vi "Main.vi"() -> ()   [LabVIEW 2018]
uses:
  <vilib>/addons/zeromq/zmq_context.lvclass
  Channel Rep/Channel Rep.lvclass
  C:/Users/orlando/Documents/Orlando/communication-manager/communication-manager/Communication Channel/Communication Channel.lvclass
  Channel Req/Channel Req.lvclass
  Channel Sub/Channel Sub.lvclass
  Channel Pub/Channel Pub.lvclass
  Communication Channel/Communication Channel.lvclass
panel:
  in  "Channel Pub.lvclass":refnum<class "Channel Pub.lvclass">
  in  "Channel Sub.lvclass":refnum<class "Channel Sub.lvclass">
  in  "Channel Req.lvclass":refnum<class "Channel Req.lvclass">
  in  "Channel Rep.lvclass":refnum<class "Channel Rep.lvclass">
  out "context":refnum<class "zmq_context.lvclass">
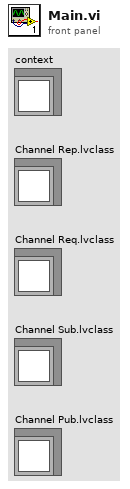
[diagram p1: front panel]
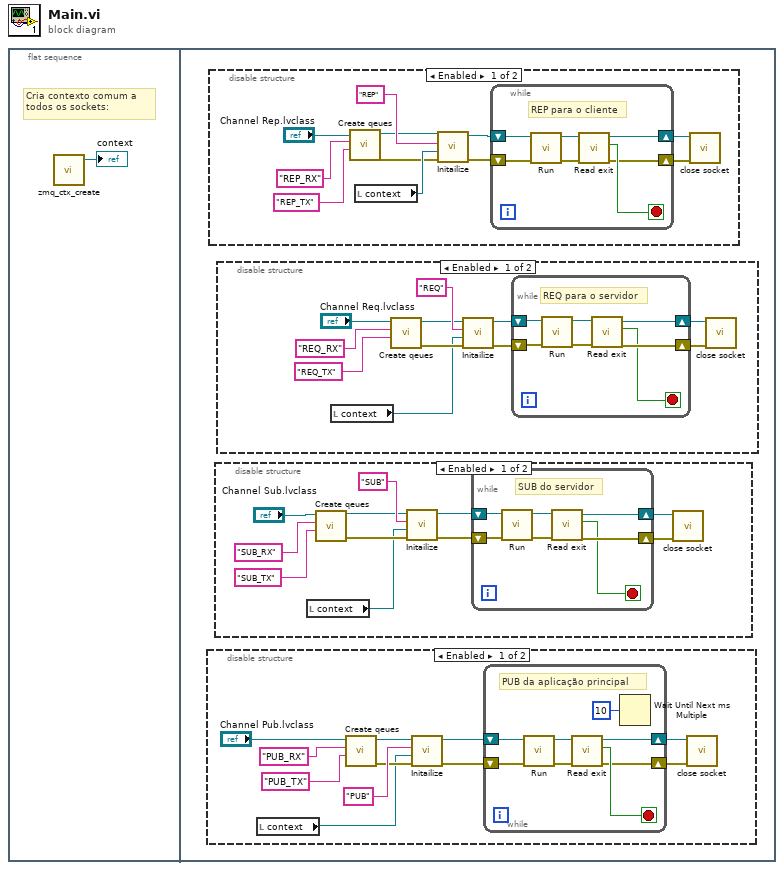
[diagram p0: block diagram]
diagram:
  n1 = flat-sequence {
    frame #0 {
      # "Cria contexto comum a \ntodos os sockets:"
      n2 = call <vilib>:"zmq_ctx_create.vi"() -> ("context out"=→"context":refnum<class "zmq_context.lvclass">)  [unwired: 4 in, 1 out]
    }
    frame #1 {
      n3 = disable-structure shown="Enabled" {
        frame Enabled {
          n4 = local read "context"() -> (w20:refnum<class "zmq_context.lvclass">)
          n5 = call "Create qeues.vi"("name qeue Tx"="PUB_TX" ("name qeue Rx"), "name qeue Rx"="PUB_RX", "Communication Channel in"="Channel Pub.lvclass") -> ("error out"=w24:errorcluster, "Communication Channel out"=w25:refnum<class "Channel Pub.lvclass">)  [unwired: 7 in]
          n6 = call-dynamic "Initailize.vi"("error in (no error)"=w24, "zeromq.lvlib:ZeroMQ Context"=w20, "Name"="PUB", "Channel Pub in"=w25) -> ("error out"=w29:errorcluster, "Channel Pub out"=w30:refnum<class "Channel Pub.lvclass">)  [unwired: 6 in]
          n7 = while {
            shift-right: [w32] -> w27
            shift-left: w30 -> [w38]
            shift-right: [w33] -> w26
            shift-left: w29 -> [w37]
            stop <- w34 stop-if-true
            # "PUB da aplicação principal"
            n8 = call-dynamic "Run.vi"("error in (no error)"=w37, "Channel Pub in"=w38) -> ("error out"=w35:errorcluster, "Channel Pub out"=w36:refnum<class "Channel Pub.lvclass">)  [unwired: 8 in]
            n9 = call-dynamic "Read exit.vi"("error in (no error)"=w35, "Communication Channel in"=w36) -> ("error out"=w33:errorcluster, "exit"=w34:bool, "Communication Channel out"=w32:refnum<class "Channel Pub.lvclass">)  [unwired: 7 in]
            n10 = Wait Until Next ms Multiple(millisecond multiple=u32 10) -> ()  [unwired: 1 out]
          }
          n11 = call "close socket.vi"("error in (no error)"=w26, "Communication Channel in"=w27) -> ()  [unwired: 8 in, 2 out]
        }
        frame Disabled {
        }
      }
      n12 = disable-structure shown="Enabled" {
        frame Enabled {
          n13 = call "Create qeues.vi"("name qeue Tx"="REP_TX" ("name qeue Rx"), "name qeue Rx"="REP_RX", "Communication Channel in"="Channel Rep.lvclass") -> ("error out"=w61:errorcluster, "Communication Channel out"=w62:refnum<class "Channel Rep.lvclass">)  [unwired: 7 in]
          n14 = local read "context"() -> (w66:refnum<class "zmq_context.lvclass">)
          n15 = call-dynamic "Initailize.vi"("error in (no error)"=w61, "zeromq.lvlib:ZeroMQ Context"=w66, "Name"="REP", "Channel Rep in"=w62) -> ("error out"=w64:errorcluster, "Channel Rep out"=w65:refnum<class "Channel Rep.lvclass">)  [unwired: 6 in]
          n16 = while {
            shift-right: [w68] -> w57
            shift-left: w65 -> [w74]
            shift-right: [w69] -> w58
            shift-left: w64 -> [w73]
            stop <- w70 stop-if-true
            # "REP para o cliente"
            n17 = call-dynamic "Run.vi"("error in (no error)"=w73, "Channel Rep in"=w74) -> ("error out"=w71:errorcluster, "Channel Rep out"=w72:refnum<class "Channel Rep.lvclass">)  [unwired: 8 in]
            n18 = call-dynamic "Read exit.vi"("error in (no error)"=w71, "Communication Channel in"=w72) -> ("error out"=w69:errorcluster, "exit"=w70:bool, "Communication Channel out"=w68:refnum<class "Channel Rep.lvclass">)  [unwired: 7 in]
          }
          n19 = call "close socket.vi"("error in (no error)"=w58, "Communication Channel in"=w57) -> ()  [unwired: 8 in, 2 out]
        }
        frame Disabled {
        }
      }
      n20 = disable-structure shown="Enabled" {
        frame Enabled {
          n21 = local read "context"() -> (w2:refnum<class "zmq_context.lvclass">)
          n22 = call "Create qeues.vi"("name qeue Tx"="SUB_TX" ("name qeue Rx"), "name qeue Rx"="SUB_RX", "Communication Channel in"="Channel Sub.lvclass") -> ("error out"=w5:errorcluster, "Communication Channel out"=w6:refnum<class "Channel Sub.lvclass">)  [unwired: 7 in]
          n23 = call-dynamic "Initailize.vi"("error in (no error)"=w5, "zeromq.lvlib:ZeroMQ Context"=w2, "Name"="SUB", "Channel Sub in"=w6) -> ("error out"=w11:errorcluster, "Channel Sub out"=w12:refnum<class "Channel Sub.lvclass">)  [unwired: 6 in]
          n24 = while {
            shift-right: [w15] -> w9
            shift-left: w12 -> [w19]
            shift-right: [w14] -> w8
            shift-left: w11 -> [w18]
            stop <- w13 stop-if-true
            # "SUB do servidor"
            n25 = call-dynamic "Run.vi"("error in (no error)"=w18, "Channel Sub in"=w19) -> ("error out"=w16:errorcluster, "Channel Sub out"=w17:refnum<class "Channel Sub.lvclass">)  [unwired: 8 in]
            n26 = call-dynamic "Read exit.vi"("error in (no error)"=w16, "Communication Channel in"=w17) -> ("error out"=w14:errorcluster, "exit"=w13:bool, "Communication Channel out"=w15:refnum<class "Channel Sub.lvclass">)  [unwired: 7 in]
          }
          n27 = call "close socket.vi"("error in (no error)"=w8, "Communication Channel in"=w9) -> ()  [unwired: 8 in, 2 out]
        }
        frame Disabled {
        }
      }
      n28 = disable-structure shown="Enabled" {
        frame Enabled {
          n29 = local read "context"() -> (w39:refnum<class "zmq_context.lvclass">)
          n30 = call "Create qeues.vi"("name qeue Tx"="REQ_TX" ("name qeue Rx"), "name qeue Rx"="REQ_RX", "Communication Channel in"="Channel Req.lvclass") -> ("error out"=w44:errorcluster, "Communication Channel out"=w45:refnum<class "Channel Req.lvclass">)  [unwired: 7 in]
          n31 = call-dynamic "Initailize.vi"("error in (no error)"=w44, "zeromq.lvlib:ZeroMQ Context"=w39, "Name"="REQ", "Channel Req in"=w45) -> ("error out"=w47:errorcluster, "Channel Req out"=w48:refnum<class "Channel Req.lvclass">)  [unwired: 6 in]
          n32 = while {
            shift-right: [w52] -> w40
            shift-left: w48 -> [w56]
            shift-right: [w51] -> w41
            shift-left: w47 -> [w55]
            stop <- w50 stop-if-true
            # "REQ para o servidor"
            n33 = call-dynamic "Run.vi"("error in (no error)"=w55, "Channel Req in"=w56) -> ("error out"=w53:errorcluster, "Channel Req out"=w54:refnum<class "Channel Req.lvclass">)  [unwired: 8 in]
            n34 = call-dynamic "Read exit.vi"("error in (no error)"=w53, "Communication Channel in"=w54) -> ("error out"=w51:errorcluster, "exit"=w50:bool, "Communication Channel out"=w52:refnum<class "Channel Req.lvclass">)  [unwired: 7 in]
          }
          n35 = call "close socket.vi"("error in (no error)"=w41, "Communication Channel in"=w40) -> ()  [unwired: 8 in, 2 out]
        }
        frame Disabled {
        }
      }
    }
  }
